vi "POP_String to Variant Value.vi"(8 "error in (no error)":errorcluster, 10 "Cell String":string, 11 "Popup Parameters":T1={"Prop Type"=enum."Unkown", "Initial Value"=variant, "Caption Strings"=[], "Ring Strings"=[], "Cell Rect"={"left"=0, "top"=0, "right"=0, "bottom"=0}, "Mouse Coords"={"x"=0, "y"=0}, "Call Data"=variant, "Ring Values"=[], "Browse Options"={"Prompt"="", "Match Pattern"="", "Mode"=enum."existing file", "Start Path"=path "", "Pattern Label"="", "Button Text"=""}, "Combo Box"={"Allow Undefined Strings"=FALSE}}) -> (0 "error out":errorcluster, 2 "Variant Value":variant, 3 "Popup Parameters out":T1={"Prop Type"=enum."Unkown", "Initial Value"=variant, "Caption Strings"=[], "Ring Strings"=[], "Cell Rect"={"left"=0, "top"=0, "right"=0, "bottom"=0}, "Mouse Coords"={"x"=0, "y"=0}, "Call Data"=variant, "Ring Values"=[], "Browse Options"={"Prompt"="", "Match Pattern"="", "Mode"=enum."existing file", "Start Path"=path "", "Pattern Label"="", "Button Text"=""}, "Combo Box"={"Allow Undefined Strings"=FALSE}})   [LabVIEW 2016]
uses:
  Ctrls/POP_Popup Call Parameters.ctl
  Ctrls/POP_Data Type.ctl
  <vilib>/Utility/miscctls.llb/LVBrowseOptionsTypeDef.ctl
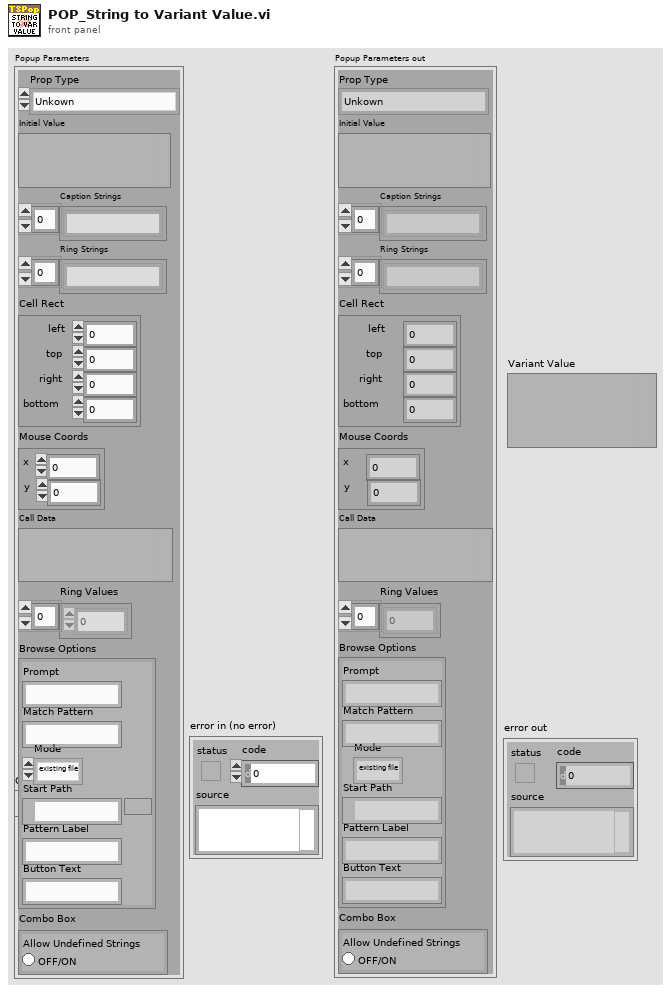
[diagram p1: front panel]
types:
  T1 = typedef "POP_Popup Call Parameters.ctl" = cluster{"Prop Type":T2, "Initial Value":variant, "Caption Strings":string[], "Ring Strings":string[], "Cell Rect":cluster{"left":i16, "top":i16, "right":i16, "bottom":i16}, "Mouse Coords":cluster{"x":i16, "y":i16}, "Call Data":variant, "Ring Values":ext[], "Browse Options":T3, "Combo Box":cluster{"Allow Undefined Strings":bool}}
  T2 = typedef "POP_Data Type.ctl" = enum16{"NO POPUP", "Unkown", "String", "Integer", "Float", "Color", "Boolean", "Ring", "Captioned String", "Captioned Integer", "Button Color", "2 Int Cluster", "4 Int Cluster", "6-Dbl Cluster", "Path", "Combox", "Time", "ShotCut String"}
  T3 = typedef "LVBrowseOptionsTypeDef.ctl" = cluster{"Prompt":string, "Match Pattern":string, "Mode":enum32{"existing file", "new file", "new or existing file", "existing dir", "new dir", "new or existing dir", "existing file (use LLBs)", "new file (use LLBs)", "new or existing file (use LLBs)", "new or existing file or directory (use LLBs)", "existing dir (use LLBs)", "new dir (use LLBs)", "new or existing dir (use LLBs)", "existing file or dir", "new file or dir", "new or existing file or dir", "existing file or dir (use LLBs)", "new file or dir (use LLBs)"}, "Start Path":path, "Pattern Label":string, "Button Text":string}
  T4 = cluster{"default value 1":i32, "default value 1":i32}
  T5 = cluster{"default value 1":i32, "default value 1":i32, "default value 1":i32, "default value 1":i32}
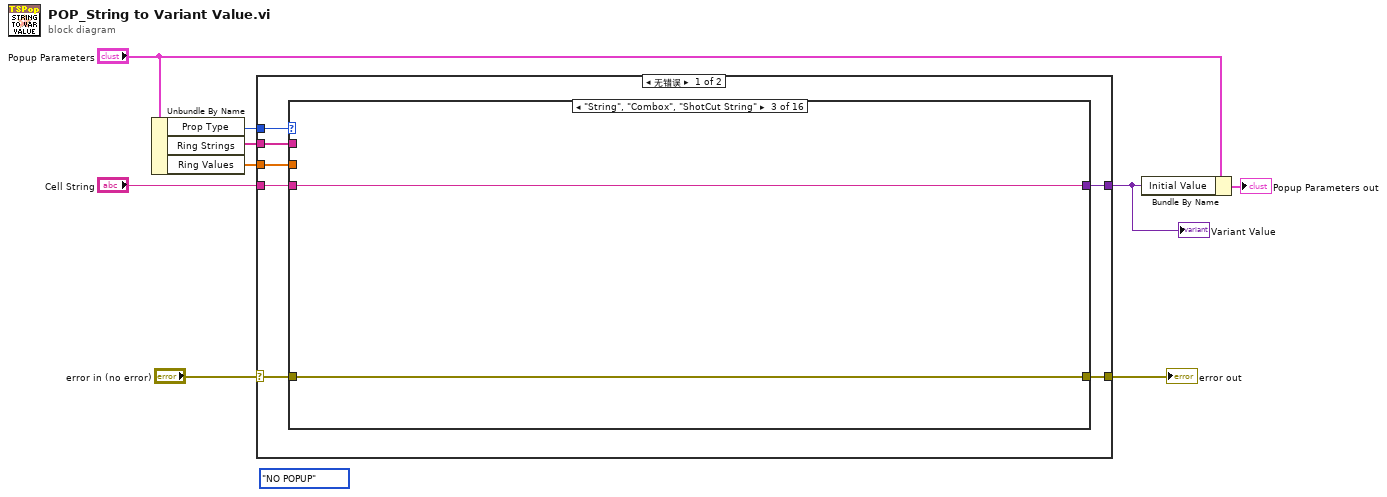
[diagram p0: block diagram]
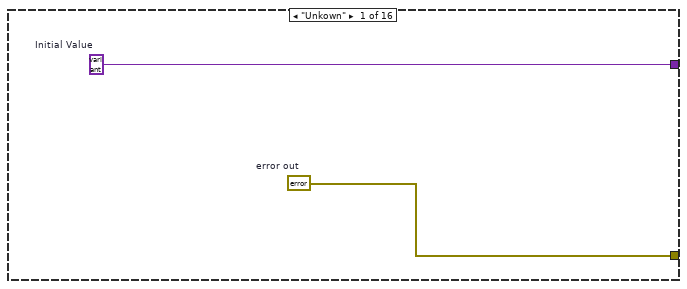
[diagram p2: hidden frame]
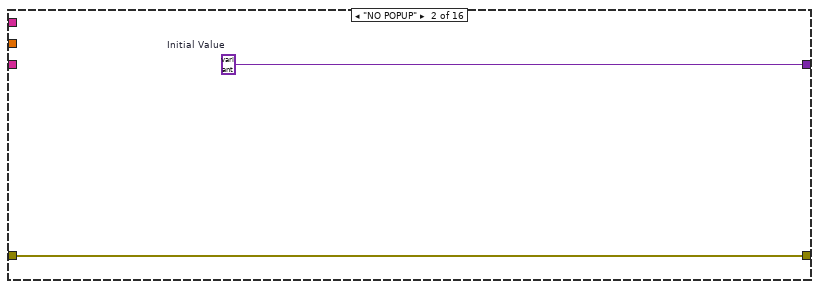
[diagram p3: hidden frame]
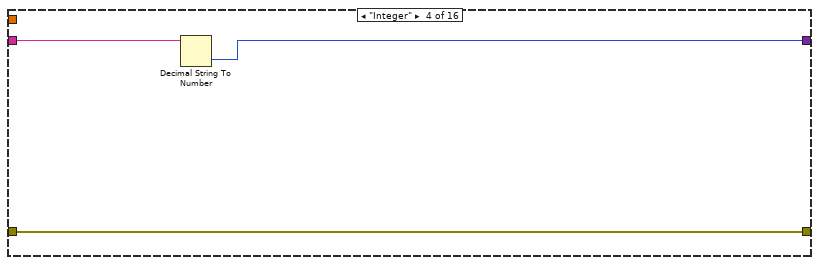
[diagram p4: hidden frame]
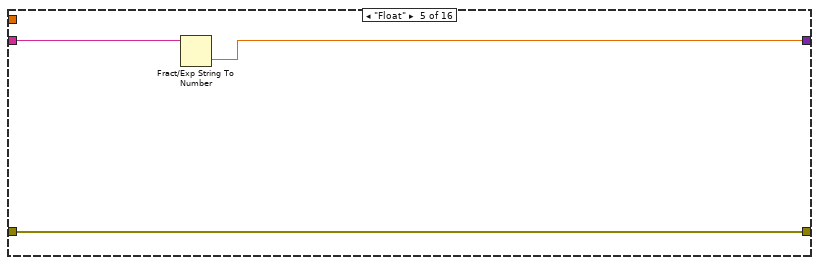
[diagram p5: hidden frame]
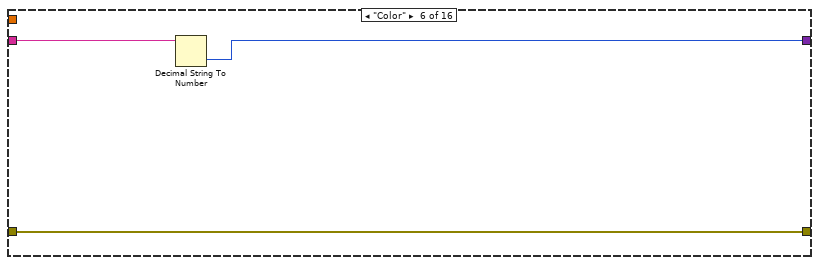
[diagram p6: hidden frame]
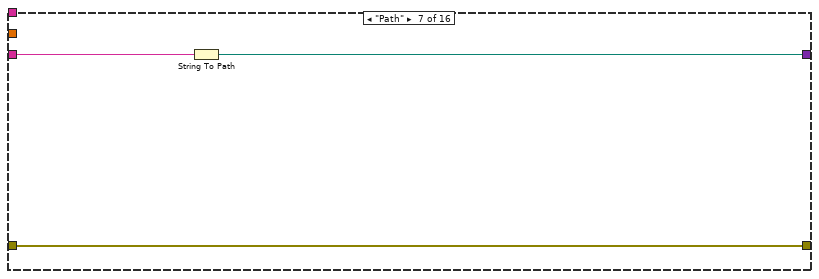
[diagram p7: hidden frame]
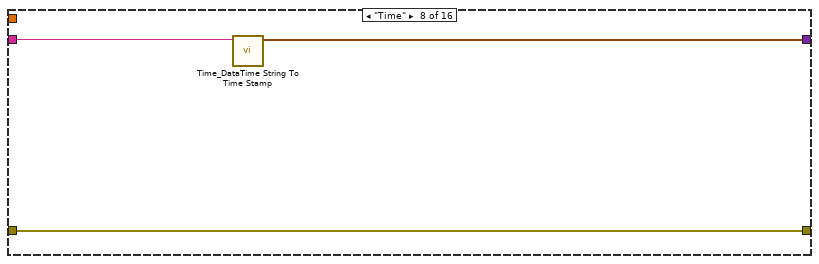
[diagram p8: hidden frame]
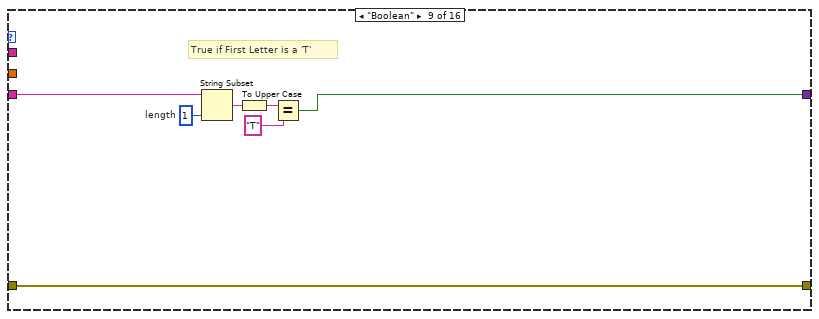
[diagram p9: hidden frame]
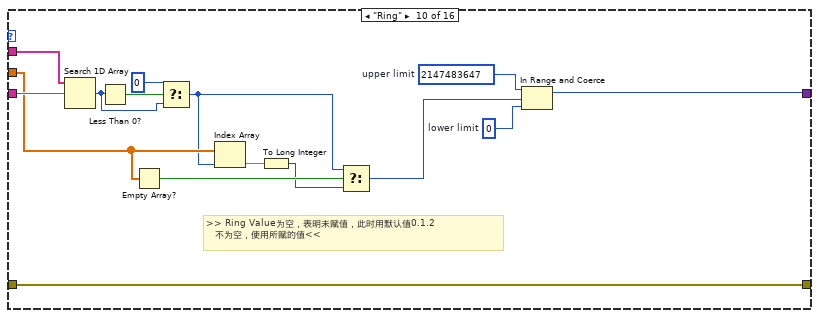
[diagram p10: hidden frame]
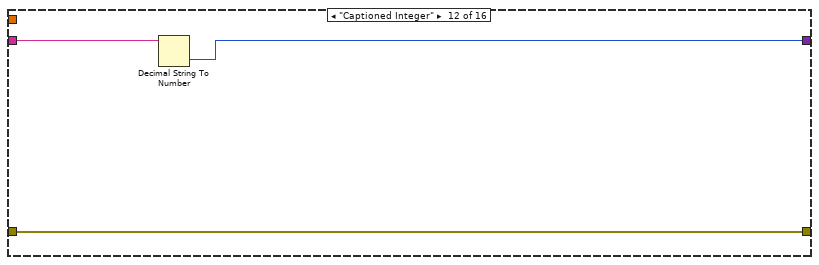
[diagram p12: hidden frame]
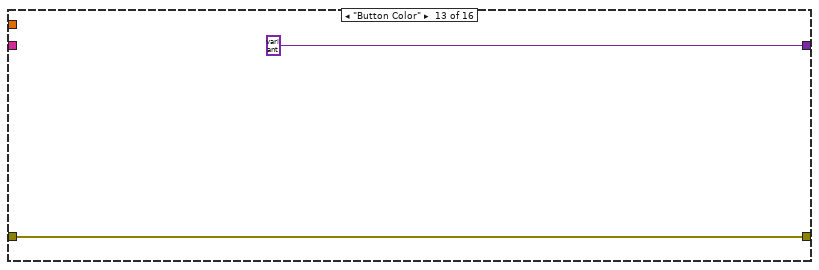
[diagram p13: hidden frame]
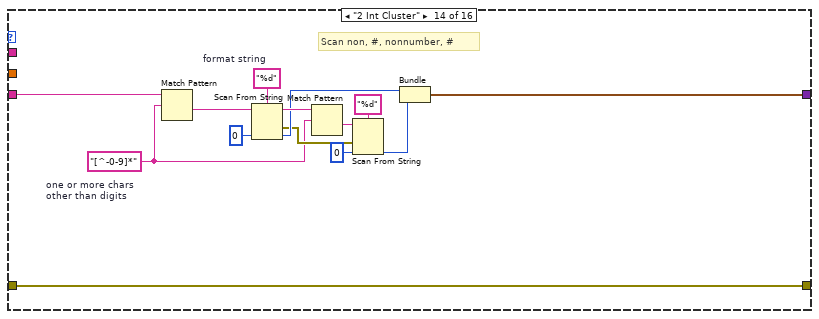
[diagram p14: hidden frame]
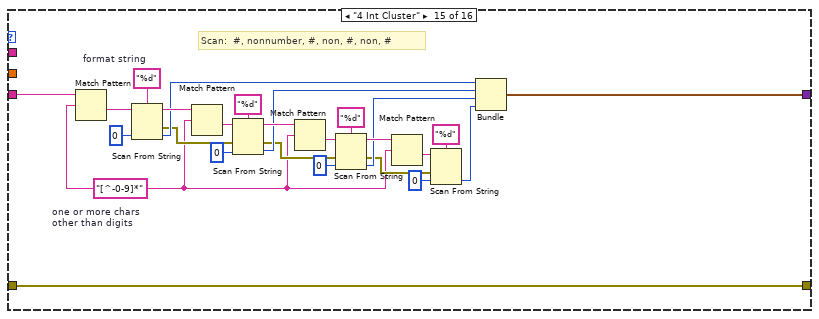
[diagram p15: hidden frame]
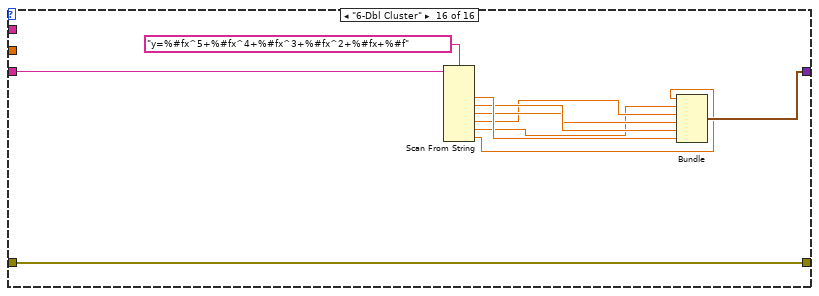
[diagram p16: hidden frame]
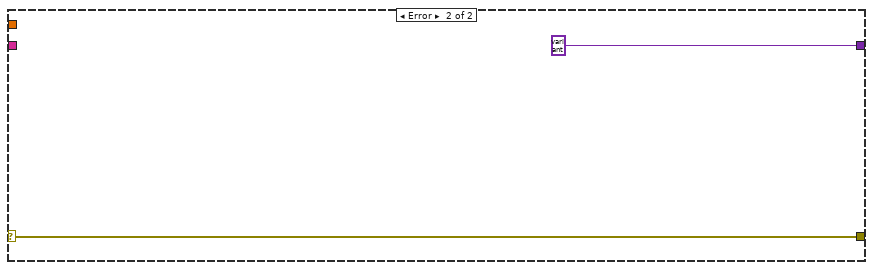
[diagram p17: hidden frame]
diagram:
  (unwired) POP_Data_Type."NO POPUP" ("Prop Type")
  n1 = Unbundle By Name("Popup Parameters") -> ("Prop Type"=w9:T2, "Ring Strings"=w6:string[], "Ring Values"=w1:ext[])
  n2 = case shown="无错误" "error in (no error)" {
    selector: "error in (no error)" -> [w13 w118]
    tunnel: w9 -> [w14 _]
    tunnel: "Cell String" -> [w16 _]
    tunnel: w6 -> [w15 _]
    tunnel: [w11 w118] -> w5
    tunnel: [w12 variant] -> w3
    tunnel: w1 -> [w10 _]
    frame No Error {
      n3 = case shown="\"String\", \"Combox\", \"ShotCut String\"" w14 {
        tunnel: [w18 w20 w22 w24 w27 w30 w32 w35 w39 w54 w61 w63 variant w73 w100 w113] -> w12
        tunnel: w16 -> [_ _ w22 w25 w28 w31 w33 w36 w44 w58 w61 w64 _ w68 w83 w114]
        tunnel: w15 -> [_ _ _ _ _ _ _ _ _ w59 _ _ _ _ _ _]
        tunnel: w13 -> [_ w19 w21 w23 w26 w29 w34 w37 w38 w57 w60 w62 w65 w70 w84 w116]
        tunnel: [w17 w19 w21 w23 w26 w29 w34 w37 w38 w57 w60 w62 w65 w70 w84 w116] -> w11
        tunnel: w10 -> [_ _ _ _ _ _ _ _ _ w52 _ _ _ _ _ _]
        frame "Unkown" {
          w17 = errorcluster {"status"=TRUE, "code"=1, "source"="Unknown Prop Type"}  # error out
          w18 = variant  # Initial Value
        }
        frame "NO POPUP" {
          w20 = variant  # Initial Value
        }
        frame "String", "Combox", "ShotCut String" {
        }
        frame "Integer" {
          n4 = Decimal String To Number(string=w25) -> (number=w24:i32)  [unwired: 2 in, 1 out]
        }
        frame "Float" {
          n5 = Fract/Exp String To Number(string=w28) -> (number=w27:dbl)  [unwired: 3 in, 1 out]
        }
        frame "Color" {
          n6 = Decimal String To Number(string=w31) -> (number=w30:i32)  [unwired: 2 in, 1 out]
        }
        frame "Path" {
          n7 = String To Path(string=w33) -> (path=w32:path)
        }
        frame "Time" {
          n8 = call "Time_DataTime String To Time Stamp.vi"("DataTime String"=w36) -> ("Time Stamp"=w35:timestamp)  [unwired: 10 in]
        }
        frame "Boolean" {
          w43 = 1  # length
          # "True if First Letter is a 'T'"
          n9 = String Subset(string=w44, length (rest)=w43) -> (substring=w42:string)  [unwired: 1 in]
          n10 = To Upper Case(1:w42) -> (0:w41:string)
          n11 = Equal?(x=w41, y="T") -> (x = y?=w39:bool)
        }
        frame "Ring" {
          w55 = 0  # lower limit
          w56 = 2147483647  # upper limit
          # ">> Ring Value为空，表明未赋值，此时用默认值0.1.2\n   不为空，使用所赋的值<<"
          n12 = Search 1D Array(1D array=w59, element=w58) -> (index of element=w45:i32)  [unwired: 1 in]
          n13 = Less Than 0?(x=w45) -> (x < 0?=w48:bool)
          n14 = Empty Array?(array=w52) -> (empty?=w51:bool)
          n15 = Select(t=0, s=w48, f=w45) -> (s? t:f=w46:i32)
          n16 = Index Array(array=w52, index=w46) -> (element=w53:ext)
          n17 = To Long Integer(number=w53) -> (32bit integer=w50:i32)
          n18 = Select(t=w46, s=w51, f=w50) -> (s? t:f=w49:i32)
          n19 = In Range and Coerce(upper limit=w56, x=w49, lower limit=w55) -> (coerced(x)=w54:i32)  [unwired: 1 out]
        }
        frame "Captioned String" {
        }
        frame "Captioned Integer" {
          n20 = Decimal String To Number(string=w64) -> (number=w63:i32)  [unwired: 2 in, 1 out]
        }
        frame "Button Color" {
        }
        frame "2 Int Cluster" {
          w67 = "[^-0-9]*"  # one or more chars other than digits
          w80 = "%d"  # format string
          # "Scan non, #, nonnumber, #"
          n21 = Match Pattern(string=w68, regular expression=w67) -> (after substring=w69:string)  [unwired: 1 in, 3 out]
          n22 = Scan From String(format string=w80, input string=w69, default 1=0 ("default value 1")) -> (remaining string=w78:string, error out=w71:errorcluster, output 1=w72:i32)  [unwired: 2 in, 1 out]
          n23 = Match Pattern(string=w78, regular expression=w67) -> (after substring=w75:string)  [unwired: 1 in, 3 out]
          n24 = Scan From String(format string="%d", input string=w75, error in=w71, default 1=0 ("default value 1")) -> (output 1=w74:i32)  [unwired: 1 in, 3 out]
          n25 = Bundle("default value 1"=w72, "default value 1"=w74) -> (w73:T4)  [unwired: 1 in]
        }
        frame "4 Int Cluster" {
          w81 = "[^-0-9]*"  # one or more chars other than digits
          w106 = "%d"  # format string
          # "Scan:  #, nonnumber, #, non, #, non, #"
          n26 = Match Pattern(string=w83, regular expression=w81) -> (after substring=w82:string)  [unwired: 1 in, 3 out]
          n27 = Scan From String(format string=w106, input string=w82, default 1=0 ("default value 1")) -> (remaining string=w104:string, error out=w87:errorcluster, output 1=w99:i32)  [unwired: 2 in, 1 out]
          n28 = Match Pattern(string=w104, regular expression=w81) -> (after substring=w101:string)  [unwired: 1 in, 3 out]
          n29 = Scan From String(format string="%d", input string=w101, error in=w87, default 1=0 ("default value 1")) -> (remaining string=w92:string, error out=w86:errorcluster, output 1=w89:i32)  [unwired: 1 in, 1 out]
          n30 = Match Pattern(string=w92, regular expression=w81) -> (after substring=w98:string)  [unwired: 1 in, 3 out]
          n31 = Scan From String(format string="%d", input string=w98, error in=w86, default 1=0 ("default value 1")) -> (remaining string=w91:string, error out=w85:errorcluster, output 1=w88:i32)  [unwired: 1 in, 1 out]
          n32 = Match Pattern(string=w91, regular expression=w81) -> (after substring=w93:string)  [unwired: 1 in, 3 out]
          n33 = Scan From String(format string="%d", input string=w93, error in=w85, default 1=0 ("default value 1")) -> (output 1=w90:i32)  [unwired: 1 in, 3 out]
          n34 = Bundle("default value 1"=w99, "default value 1"=w89, "default value 1"=w88, "default value 1"=w90) -> (w100:T5)  [unwired: 1 in]
        }
        frame "6-Dbl Cluster" {
          n35 = Scan From String(format string="y=%#fx^5+%#fx^4+%#fx^3+%#fx^2+%#fx+%#f", input string=w114) -> (output 1=w112:dbl, output 2=w111:dbl, output 3=w110:dbl, output 4=w109:dbl, output 5=w108:dbl, output 6=w107:dbl)  [unwired: 8 in, 3 out]
          n36 = Bundle(w107, w108, w109, w110, w111, w112) -> (w113:cluster{dbl, dbl, dbl, dbl, dbl, dbl})  [unwired: 1 in]
        }
      }
    }
    frame Error {
    }
  }
  "error out" <- w5
  "Variant Value" <- w3
  n37 = Bundle By Name(cluster="Popup Parameters", "Initial Value"=w3) -> (→"Popup Parameters out":T1)
